vi "Init Control.vi"(5 "Group":refnum<class "Group.lvclass">, 6 "Period ms":i64, 7 "VolatusAPI":refnum<class "VolatusAPI.lvclass">, 8 "error in (no error)":errorcluster, 9 "Control MsgQ":refnum<class "MessageQ.lvclass">, 10 "Config Element":refnum<class "Config Element.lvclass">, 11 "Valve in":refnum<class "ValueSetControl.lvclass">) -> (0 "error out":errorcluster, 3 "Valve out":refnum<class "ValueSetControl.lvclass">)   [LabVIEW 2020, in "VolatusControl.lvlib" / "ValueSetControl.lvclass"]
uses:
  ValueSetControl.lvclass
  ValueSetControl.lvclass/ValueSetControl.ctl
  lv-cdm/CDM-Config/Config Element/Config Element.lvclass
  Volatus/VolatusAPI/VolatusAPI.lvclass
  lv-vecto/Vecto/GroupAbstract/GroupAbstract.lvclass
  lv-vecto/Vecto/Group/Group.lvclass
  C:/dev/lv20CE/relink/lv-vecto/Vecto/GroupAbstract/GroupAbstract.lvclass
  C:/dev/lv20CE/relink/lv-vecto/Vecto/Group/Group.lvclass
  Volatus/MessageQ/MessageQ.lvclass
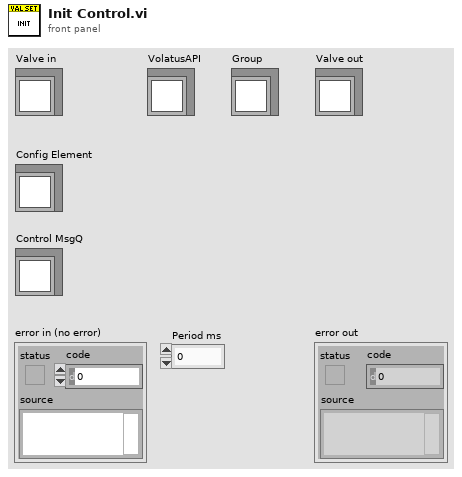
[diagram p1: front panel]
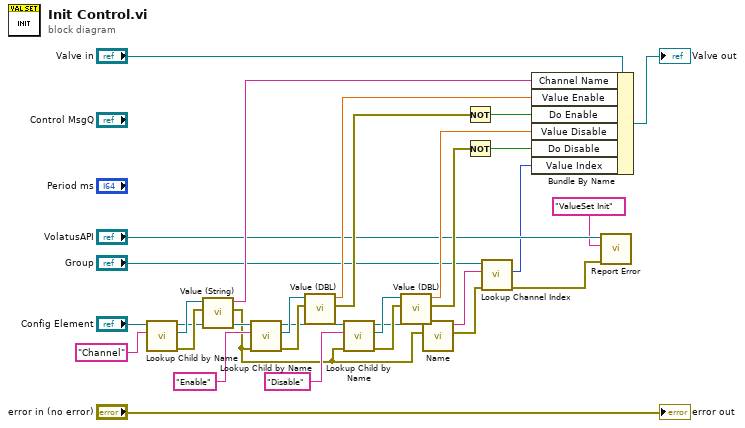
[diagram p0: block diagram]
diagram:
  n1 = call "Lookup Child by Name.vi"("Name"="Channel", "Config Element in"="Config Element") -> ("error out"=w25:errorcluster, "Child"=w26:refnum<class "Config Element.lvclass">, "Config Element out"=w23:refnum<class "Config Element.lvclass">)  [unwired: 6 in, 1 out]
  n2 = call "Value (String).vi"("error in (no error)"=w25, "Config Element in"=w26) -> ("error out"=w6:errorcluster, "String Value"=w24:string)  [unwired: 8 in]
  n3 = call "Lookup Child by Name.vi"("error in (no error)"=w6, "Name"="Enable", "Config Element in"=w23) -> ("error out"=w20:errorcluster, "Child"=w21:refnum<class "Config Element.lvclass">, "Config Element out"=w18:refnum<class "Config Element.lvclass">)  [unwired: 5 in, 1 out]
  n4 = call "Value (DBL).vi"("error in (no error)"=w20, "Config Element in"=w21) -> ("error out"=w10:errorcluster, "DBL Value"=w19:dbl)  [unwired: 8 in]
  n5 = call "Lookup Child by Name.vi"("error in (no error)"=w6, "Name"="Disable", "Config Element in"=w18) -> ("error out"=w15:errorcluster, "Child"=w16:refnum<class "Config Element.lvclass">, "Config Element out"=w7:refnum<class "Config Element.lvclass">)  [unwired: 5 in, 1 out]
  n6 = call "Value (DBL).vi"("error in (no error)"=w15, "Config Element in"=w16) -> ("error out"=w11:errorcluster, "DBL Value"=w14:dbl)  [unwired: 8 in]
  n7 = call "Name.vi"("error in (no error)"=w6, "Config Element in"=w7) -> ("error out"=w5:errorcluster, "Name"=w2:string)  [unwired: 8 in]
  n8 = Not(x=w10) -> (.not. x?=w13:bool)
  n9 = Not(x=w11) -> (.not. x?=w12:bool)
  n10 = call "Lookup Channel Index.vi"("error in (no error)"=w5, "Channel Name"=w2, "GroupAbstract in"="Group") -> ("error out"=w4:errorcluster, "Index"=w1:i32)  [unwired: 6 in, 1 out]
  n11 = Bundle By Name(cluster="Valve in", "Channel Name"=w24, "Value Enable"=w19, "Do Enable"=w13, "Value Disable"=w14, "Do Disable"=w12, "Value Index"=w1) -> (→"Valve out":refnum<class "ValueSetControl.lvclass">)
  n12 = call "Report Error.vi"("error in (no error)"=w4, "Context"="ValueSet Init", "VolatusAPI in"="VolatusAPI") -> ()  [unwired: 7 in, 2 out]
  "error out" <- "error in (no error)"
